vi "EJ 4.1.4.vi"() -> ()   [LabVIEW 2013]
uses:
  <vilib>/gmath/statdist.llb/Normal Inverse CDF.vi
  <vilib>/gmath/NI_Gmath.lvlib
panel:
  out "Waveform Chart":cluster{"x":dbl, dbl}(graph)
  in  "stop":bool
  in  "Nivel de ruido":dbl
  in  "Medicion":dbl
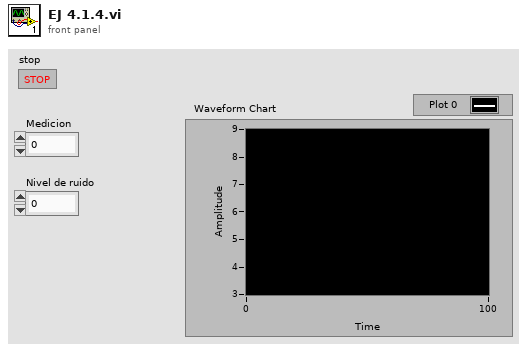
[diagram p1: front panel]
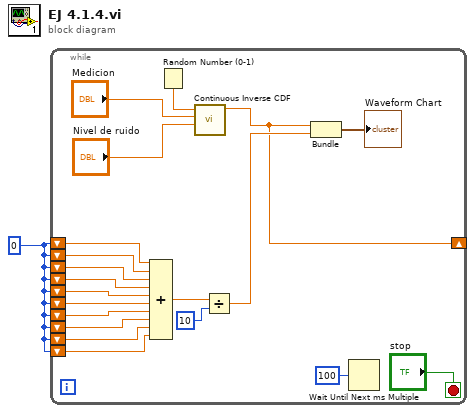
[diagram p0: block diagram]
diagram:
  w1 = 0
  n1 = while {
    shift-right: [w2] -> _
    shift-left: w1 -> [w14]
    shift-left: w1 -> [w13]
    shift-left: w1 -> [w12]
    shift-left: w1 -> [w11]
    shift-left: w1 -> [w10]
    shift-left: w1 -> [w9]
    shift-left: w1 -> [w8]
    shift-left: w1 -> [w7]
    shift-left: w1 -> [w15]
    shift-left: w1 -> [w16]
    stop <- "stop" stop-if-true
    n2 = Compound Arithmetic op=ADD(w16, w15, w14, w13, w12, w11, w10, w9, w8, w7) -> (w6:dbl)
    n3 = Random Number (0-1)() -> (number: 0 to 1=w17:dbl)
    n4 = call-poly <vilib>:"Continuous Inverse CDF.vi"("std"="Nivel de ruido", "mean"="Medicion", "cdf(x)"=w17) -> ("x"=w2:dbl)  [unwired: 7 in, 1 out]
    n5 = Divide(x=w6, y=10) -> (x/y=w3:dbl)
    n6 = Bundle("x"=w2, w3) -> (→"Waveform Chart":cluster{"x":dbl, dbl})  [unwired: 1 in]
    n7 = Wait Until Next ms Multiple(millisecond multiple=u32 100) -> ()  [unwired: 1 out]
  }
